vi "Perf Read Data.vi"(8 "error in (no error)":errorcluster) -> (0 "error out":errorcluster, 3 "Performance Data":T1)   [LabVIEW 2017, in "Performance.lvlib"]
uses:
  Performance.lvlib
  Private FGV/Performance Data.ctl
  Dependencies/lv_system_tools/lv_system_tools_100/tools_system CPU Usage Ref.ctl
  Private FGV/Performance Methods.ctl
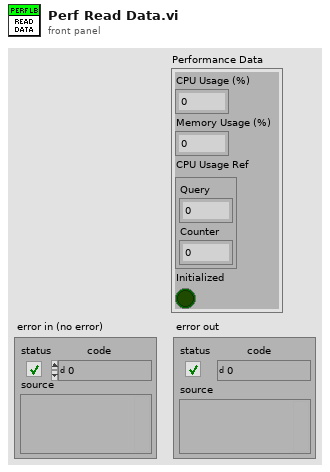
[diagram p1: front panel]
types:
  T1 = typedef "Performance.lvlib/Performance Data.ctl" = cluster{"CPU Usage (%)":dbl, "Memory Usage (%)":dbl, "CPU Usage Ref":T2, "Initialized":bool}
  T2 = typedef "Performance.lvlib/tools_system CPU Usage Ref.ctl" = cluster{"Query":u32, "Counter":u32}
  T3 = typedef "Performance.lvlib/Performance Methods.ctl" = enum16{"Init", "Get Data", "Close"}
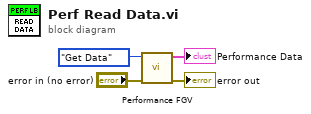
[diagram p0: block diagram]
diagram:
  n1 = call "Performance FGV.vi"("error in (no error)"="error in (no error)", "Performance Methods"=Performance_Methods."Get Data") -> ("error out"=→"error out":errorcluster, "Performance Data"=→"Performance Data":T1)  [unwired: 8 in]
